vi "Exit.vi"(8 "error in (no error)":errorcluster, 11 "Idle in":refnum<class "Idle.lvclass">) -> (0 "error out":errorcluster, 3 "Idle out":refnum<class "Idle.lvclass">)   [LabVIEW 2014, in "States.lvlib" / "Idle.lvclass"]
doc: "This override sends a Log Event message to the UI, with the string \"Exiting Idle State\" as its payload."
uses:
  Idle.lvclass
  <vilib>/ActorFramework/Actor/Actor.lvclass/Actor.ctl
  labview/1512/State Pattern Actor Example/State Pattern UI/Log Event Msg/Log Event Msg.lvclass/Log Event Msg.ctl
  <vilib>/ActorFramework/Message Enqueuer/Message Enqueuer.lvclass/Message Enqueuer.ctl
  <vilib>/ActorFramework/Message Enqueuer/Enqueue.vi
  <vilib>/ActorFramework/Message Priority Queue/Priority Enqueue.vi
  Process State/Process State.lvclass
  labview/1512/State Pattern Actor Example/State Pattern UI/Log Event Msg/Log Event Msg.lvclass
  <vilib>/ActorFramework/Actor/Actor.lvclass
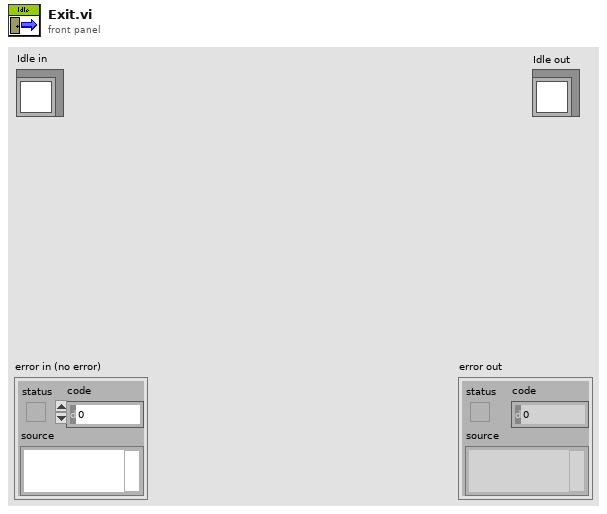
[diagram p1: front panel]
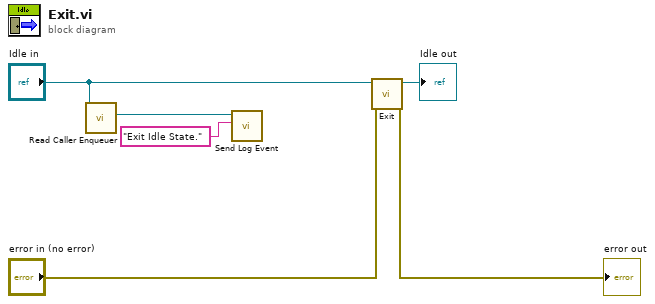
[diagram p0: block diagram]
diagram:
  n1 = call <vilib>:"Read Caller Enqueuer.vi"("Actor"="Idle in") -> ("Caller Enqueuer"=w6:refnum<class "Message Enqueuer.lvclass">)  [unwired: 10 in]
  n2 = call "Send Log Event.vi"("Event Text"="Exit Idle State.", "Message Enqueuer"=w6) -> ()  [unwired: 9 in, 1 out]
  n3 = call-parent "Exit.vi"("error in (no error)"="error in (no error)", "Old State"="Idle in") -> ("error out"=→"error out":errorcluster, "New State"=→"Idle out":refnum<class "Idle.lvclass">)  [unwired: 8 in]
